vi "myRIO_BRig_RT_dataExp_Audio_freq__R.vi"() -> (2 "output_Audio_freq__R":i32)   [LabVIEW 2014]
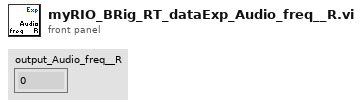
[diagram p1: front panel]
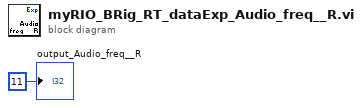
[diagram p0: block diagram]
diagram:
  "output_Audio_freq__R" <- 11 ("output_iBlock")
